vi "Speed to Delay.vi"(9 "max delay":dbl=500.0 format="%#_13g", 10 "min delay":dbl format="%#_13g", 11 "Speed":dbl) -> (3 "upper limit":dbl)   [LabVIEW 2015]
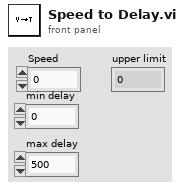
[diagram p1: front panel]
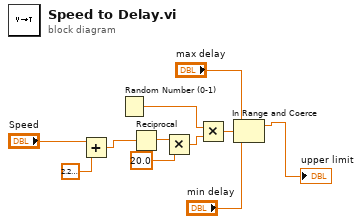
[diagram p0: block diagram]
diagram:
  n1 = Add(x="Speed", y=2.220446049250313e-16) -> (x+y=w7:dbl)
  n2 = Random Number (0-1)() -> (number: 0 to 1=w4:dbl)
  n3 = Reciprocal(x=w7) -> (1/x=w1:dbl)
  n4 = Multiply(x=w1, y=20.0) -> (x*y=w3:dbl)
  n5 = Multiply(x=w4, y=w3) -> (x*y=w8:dbl)
  n6 = In Range and Coerce(upper limit="max delay", x=w8, lower limit="min delay") -> (coerced(x)=→"upper limit":dbl)  [unwired: 1 out]
